vi "decimate.vi"(9 "offset":u16, 10 "decimation":u16, 11 "run flags":u8) -> (1 "new offset":u16, 2 "decimation out":u16, 3 "run flags out":u8)   [LabVIEW 2013, in "main engine.lvlib"]
uses:
  main engine/main engine.lvlib
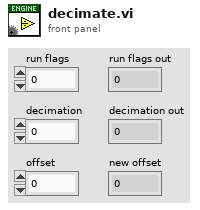
[diagram p1: front panel]
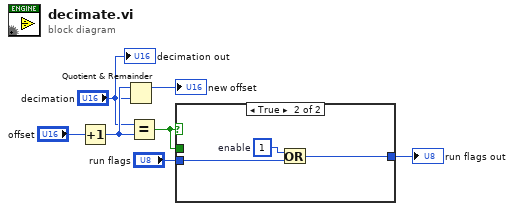
[diagram p0: block diagram]
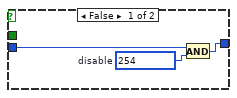
[diagram p2: hidden frame]
diagram:
  n1 = Increment(x="offset") -> (x+1=w6:u16)
  n2 = Quotient & Remainder(x=w6, y="decimation") -> (x-y*floor(x/y)=→"new offset":u16)  [unwired: 1 out]
  n3 = Equal?(x="decimation", y=w6) -> (x = y?=w1:bool)
  n4 = case shown="True" w1 {
    tunnel: w1 -> [_ _]
    tunnel: "run flags" -> [w10 w13]
    tunnel: [w8 w11] -> w2
    frame False {
      w9 = u8 254  # disable
      n5 = And(x=w10, y=w9) -> (x .and. y?=w8:u8)
    }
    frame True {
      w12 = u8 1  # enable
      n6 = Or(x=w12, y=w13) -> (x .or. y?=w11:u8)
    }
  }
  "run flags out" <- w2
  "decimation out" <- "decimation"
